vi "niRFUtil RFHS FIFO Delete.vi"(0 "Fifo ID":T1, 11 "error in (no error)":errorcluster) -> (15 "error out":errorcluster)   [LabVIEW 2015, in "niRFUtil.lvlib"]
uses:
  niRFUtil.lvlib
  niRFUtil RFHS FIFO Reference.ctl
  niRFUtil RFHS FIFO.ctl
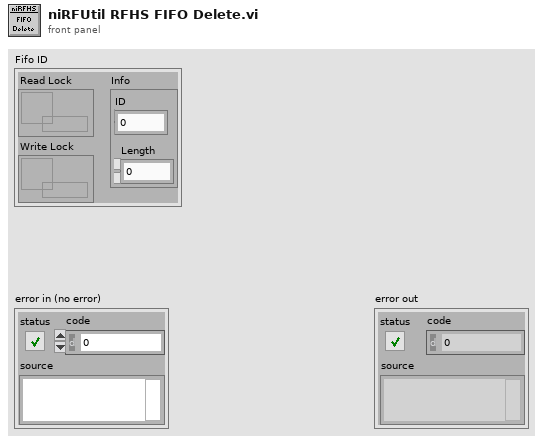
[diagram p1: front panel]
types:
  T1 = typedef "niRFUtil.lvlib/niRFUtil RFHS FIFO Reference.ctl" = cluster{"Read Lock":refnum<data-value>, "Info":T2, "Write Lock":refnum<data-value>}
  T2 = typedef "niRFUtil.lvlib/niRFUtil RFHS FIFO.ctl" = cluster{"ID":u64, "Length":u32}
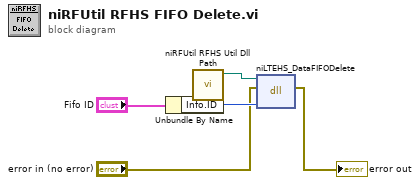
[diagram p0: block diagram]
diagram:
  n1 = Unbundle By Name("Fifo ID") -> ("Info.ID"=w3:u64)
  n2 = call "niRFUtil RFHS Util Dll Path.vi"() -> ("Path"=w5:path)  [unwired: 7 in, 4 out]
  n3 = dll-call lib="C:/Users/avrancic.000/Documents/_NI/RF/LTE Turbo Stuff/niLTE/trunk/source/Labview/common/niLTE.dll" fn="niLTEHS_DataFIFODelete"(path in=w5, error in="error in (no error)", "fifoId"=w3) -> (error out=→"error out":errorcluster)  [unwired: 3 in, 1 out]
